vi "Keep time (SubVI).vi"(10 "Injection":bool, 11 "Time Target (s)":dbl) -> (2 "Measurement running?":bool, 3 "Elapsed Time (s)":dbl)   [LabVIEW 2014]
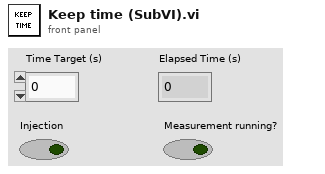
[diagram p1: front panel]
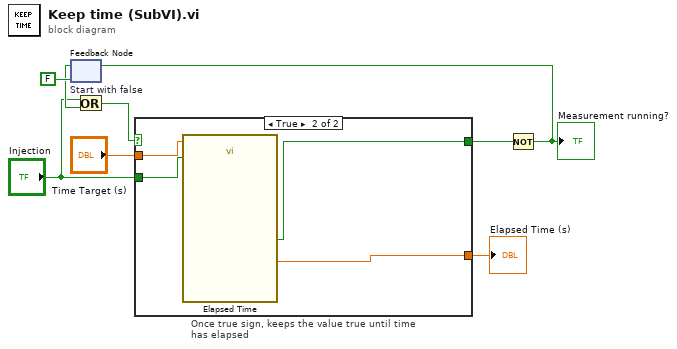
[diagram p0: block diagram]
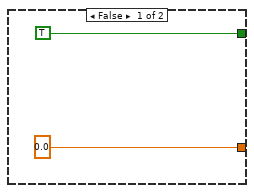
[diagram p2: hidden frame]
diagram:
  n1 = feedback #1 "Start with false"(FALSE) -> (w2:bool)
  n2 = Or(x="Injection", y=w2) -> (x .or. y?=w5:bool)
  n3 = case "Once true sign, keeps the value true until time has elapsed" shown="True" w5 {
    tunnel: "Time Target (s)" -> [_ w14]
    tunnel: [0.0 ("Elapsed Time (s)") w13] -> w7
    tunnel: [TRUE ("Time has Elapsed") w12] -> w8
    tunnel: "Injection" -> [_ w11]
    frame False {
    }
    frame True {
      n4 = call "Elapsed Time"("Time Target (s)"=w14, "Reset"=w11) -> ("Elapsed Time (s)"=w13:dbl, "Time has Elapsed"=w12:bool)  [unwired: 10 in, 6 out]
    }
  }
  "Elapsed Time (s)" <- w7
  n5 = Not(x=w8) -> (.not. x?=w3:bool)
  "Measurement running?" <- w3
  n6 = feedback-in #1(w3) -> ()
